vi "mkConfigure.vi"(10 "Camera in":T1={"Gain [1-4]"=10.0, "Offset"=1, "Mode"=75, "ROIs"=[], "ROI Size"={"X"=0, "Y"=0}, "Number of buffers"=40, "Use hardware multiple-ROI?"=TRUE, "GenericCameraConfig"={"Framerate (Hz)"=60, "Exposure time (us)"=5000, "Image size"={"Width"=1280, "Height"=1024}, "Number of buffers"=30}}, 11 "IMAQ Session":refnum<k11>) -> (3 "IMAQ Refnum out":refnum<k11>, 7 "Camera Mode [out]":i32)   [LabVIEW 2011]
uses:
  CameraConfig.ctl
  Main/Camera/GenericCameraConfigType.ctl
panel:
  # "us"
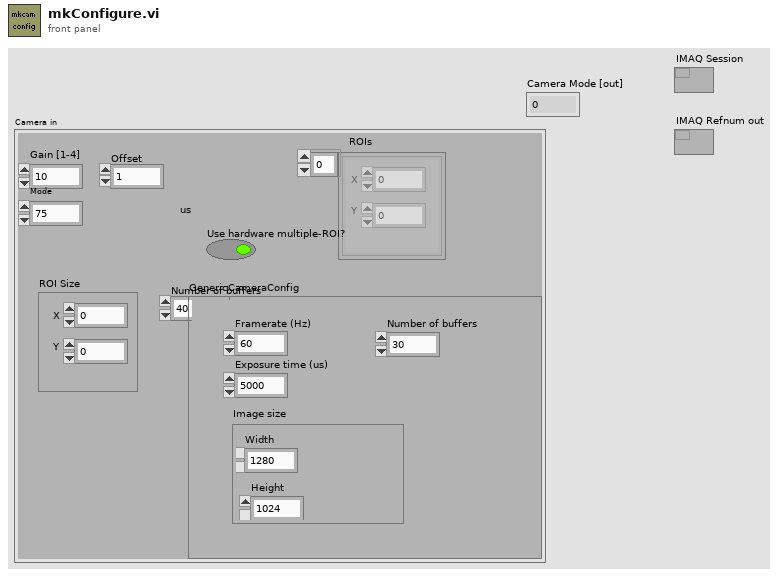
[diagram p1: front panel]
types:
  T1 = typedef "CameraConfig.ctl" = cluster{"Gain [1-4]":sgl, "Offset":i16, "Mode":i16, "ROIs":cluster{"X":i32, "Y":i32}[], "ROI Size":cluster{"X":i32, "Y":i32}, "Number of buffers":i32, "Use hardware multiple-ROI?":bool, "GenericCameraConfig":T2}
  T2 = typedef "GenericCameraConfigType.ctl" = cluster{"Framerate (Hz)":i32, "Exposure time (us)":i32, "Image size":cluster{"Width":i32, "Height":i32}, "Number of buffers":i32}
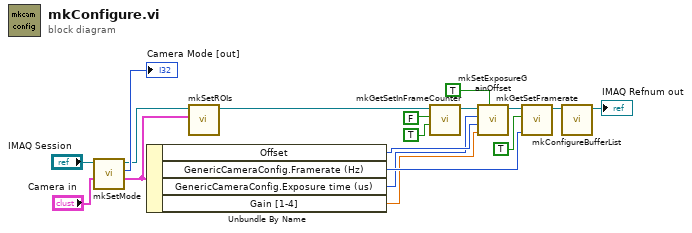
[diagram p0: block diagram]
diagram:
  n1 = call "mkSetMode.vi"("Camera in"="Camera in", "IMAQ Refnum in"="IMAQ Session") -> ("Camera Settings"=w3:T1, "Camera Mode [out]"=→"Camera Mode [out]":i32, "IMAQ Refnum out"=w12:refnum<k11>)  [unwired: 7 in]
  n2 = Unbundle By Name(w3) -> ("Offset"=w5:i16, "GenericCameraConfig.Framerate (Hz)"=w16:i32, "GenericCameraConfig.Exposure time (us)"=w4:i32, "Gain [1-4]"=w6:sgl)
  n3 = call "mkSetROIs.vi"("Camera in"=w3, "IMAQ Refnum in"=w12) -> ("IMAQ Refnum out"=w2:refnum<k11>)  [unwired: 9 in]
  n4 = call "mkGetSetInFrameCounter.vi"("Set? (F)"=TRUE, "Enable in-frame counter (T)"=FALSE, "IMAQ Refnum in"=w2) -> ("IMAQ Refnum out"=w7:refnum<k11>)  [unwired: 7 in, 1 out]
  n5 = call "mkSetExposureGainOffset.vi"("Set? (F)"=TRUE, "Gain [1-4]"=w6, "Offset"=w5, "Exposure time"=w4, "IMAQ Refnum in"=w7) -> ("IMAQ Refnum out"=w17:refnum<k11>)  [unwired: 1 in, 5 out]
  n6 = call "mkGetSetFramerate.vi"("Framerate"=w16, "Set? (F)"=TRUE, "IMAQ Refnum out"=w17) -> ("IMAQ Refnum (out)"=w1:refnum<k11>)  [unwired: 5 in, 3 out]
  n7 = call "mkConfigureBufferList.vi"("IMAQ Session"=w1) -> ("IMAQ Session (out)"=→"IMAQ Refnum out":refnum<k11>)  [unwired: 10 in]
